vi "LIA FFT Refreseher.vi"() -> ()   [LabVIEW 2017]
uses:
  <vilib>/Analysis/2dsp.llb/Real FFT.vi
  <vilib>/Analysis/NI_AALBase.lvlib
  <vilib>/Analysis/NI_AALPro.lvlib
panel:
  in  "offset":dbl=1.0 format="%0.2f"
  out "Waveform Graph 2":dbl[](graph)
  in  "cycles":dbl=1.0 format="%0.2f"
  out "Waveform Graph 1":dbl[](graph)
  in  "amplitude":dbl=1.0 format="%0.2f"
  in  "samples":i32=128
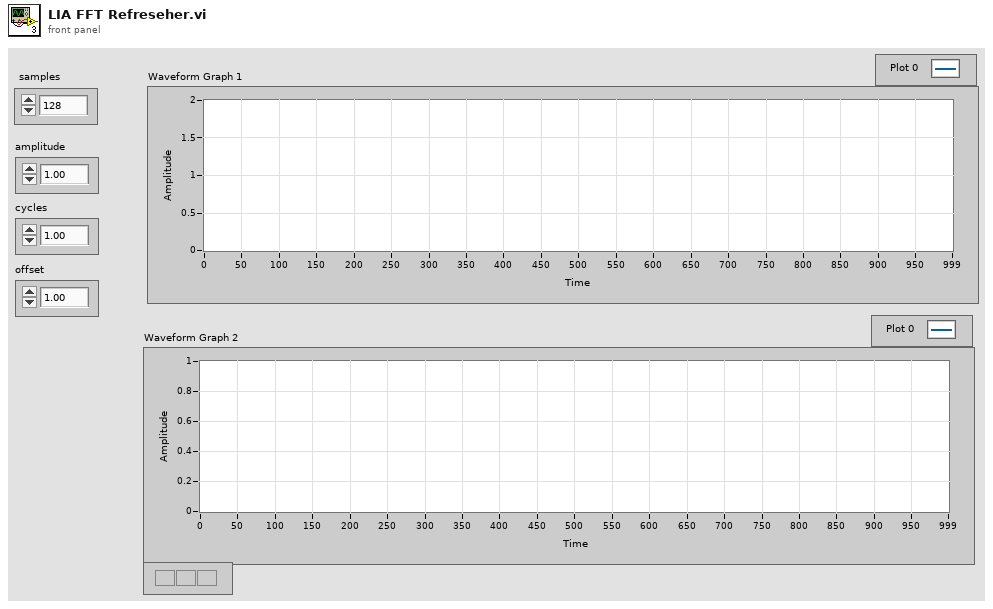
[diagram p1: front panel]
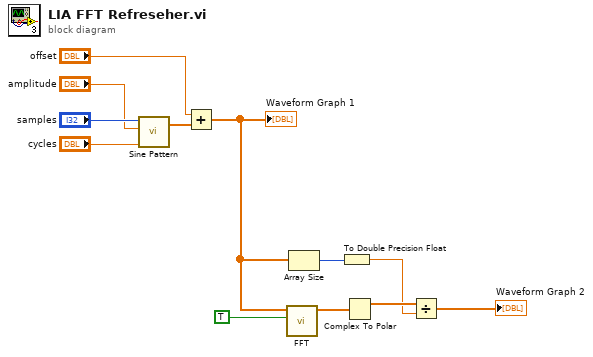
[diagram p0: block diagram]
diagram:
  n1 = call <vilib>:"Sine Pattern.vi"("cycles"="cycles", "amplitude"="amplitude", "samples"="samples") -> ("Sinusoidal Pattern"=w5:dbl[])  [unwired: 1 in, 1 out]
  n2 = Add(x="offset", y=w5) -> (x+y=w2:dbl[])
  "Waveform Graph 1" <- w2
  n3 = call-poly <vilib>:"FFT.vi"("shift?"=TRUE, "X"=w2) -> ("FFT {X}"=w9:cdb[])  [unwired: 8 in, 1 out]
  n4 = Array Size(array=w2) -> (size(s)=w4:i32)
  n5 = To Double Precision Float(number=w4) -> (double precision float=w3:dbl)
  n6 = Complex To Polar(r * e^(i*theta)=w9) -> (r=w6:dbl[])  [unwired: 1 out]
  n7 = Divide(x=w6, y=w3) -> (x/y=→"Waveform Graph 2":dbl[])
